vi "Read Port Names.vi"(8 "error in (no error)":errorcluster, 11 "Cal Standard Sim in":refnum<class "Cal Standard Sim.lvclass">) -> (0 "error out":errorcluster, 2 "Port Names":string[](array[string]), 3 "Cal Standard Sim out":refnum<class "Cal Standard Sim.lvclass">)   [LabVIEW 2023, in "RFFixtureCharact.Instruments.lvlib" / "Cal Standard Sim.lvclass"]
uses:
  Cal Standard Sim.lvclass
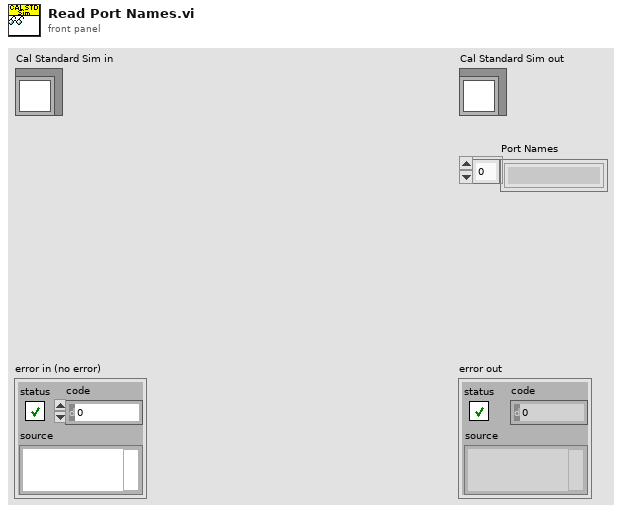
[diagram p1: front panel]
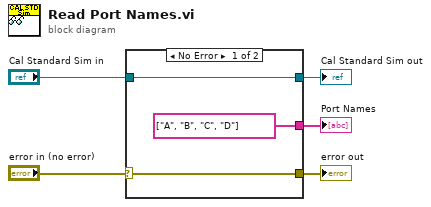
[diagram p0: block diagram]
diagram:
  n1 = case shown="No Error" "error in (no error)" {
    selector: "error in (no error)" -> [w8 w9]
    tunnel: [w8 w9] -> w5
    tunnel: [w7 w10] -> w4
    tunnel: "Cal Standard Sim in" -> [w7 w10]
    tunnel: [string[] ["A", "B", "C", "D"] ("ACM4509 Port Names") _] -> w1
    frame No Error {
    }
    frame Error {
    }
  }
  "error out" <- w5
  "Cal Standard Sim out" <- w4
  "Port Names" <- w1
